vi "WindowOccluded.vi"(8 "error in (no error)":errorcluster, 10 "Timestamp":u64, 11 "WindowEventInterface in":refnum<class "WindowEventInterface.lvclass">) -> (0 "error out":errorcluster)   [LabVIEW 2020, in "GLF.lvlib" / "WindowEventInterface.lvclass"]
uses:
  WindowEventInterface.lvclass
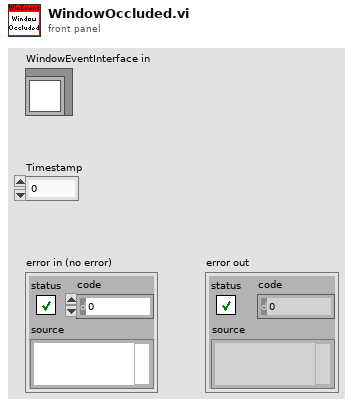
[diagram p1: front panel]
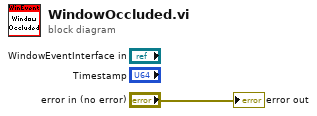
[diagram p0: block diagram]
diagram:
  "error out" <- "error in (no error)"
